vi "glueing_proc_switch_3cartucce.vi"() -> ()   [LabVIEW 2011]
panel:
  in  "Start 3":bool
  in  "spint down - III part":bool
  in  "glue press 2mm - III part":bool
  in  "spint down - III part":bool
  in  "zero Spint for replacing glue 2":bool
  in  "KILL":bool
  in  "PAUSE":bool
  in  "RESUME":bool
  in  "QUIT":bool
  in  "goto y pos":bool
  in  "goto x pos":bool
  in  "Tavolo o stiffback?":bool
  in  "fine tuning y \nmove +2 mm":bool
  in  "fine tuning x \nmove - 2 mm":bool
  in  "fine tuning y \nmove - 2 mm":bool
  in  "fine tuning x \nmove + 2 mm":bool
  in  "Start 2":bool
  in  "spint down - II part":bool
  in  "glue press 2mm - II part":bool
  in  "spint down - II part":bool
  in  "zero done 2":bool
  in  "zero Gluer - end":bool
  in  "zero x - end":bool
  in  "zero y - end":bool
  in  "zero Spint - end":bool
  in  "zero Spint for replacing glue":bool
  in  "spint down 2":bool
  in  "glue press 2mm":bool
  in  "spint down":bool
  in  "Start":bool
  in  "fine tuning z dw 1mm":bool
  in  "fine tuning z up 1mm":bool
  in  "goto z pos 2":bool
  in  "goto z pos":bool
  in  "positioning done":bool
  in  "zero Spint":bool
  out "output":string
  out "command":string
  in  "zero done":bool
  in  "zero Gluer":bool
  in  "zero x":bool
  in  "zero y":bool
  # "In alto: TRUE ---> TAVOLO\nIn basso: FALSE ---> STIFFBACK"
  # "Posiziono in zero"
  # "Vado in posizione"
  # "Fine tuning in posizione x e y \nsolo se necessario"
  # "Muovo spintore e inizio a incollare"
  # "Cambio cartuccia della colla\n\nSTART riprende incollaggio"
  # "Cambio cartuccia della colla\n\nSTART riprende incollaggio"
  # "Scarico la colla e \nritorno a zero"
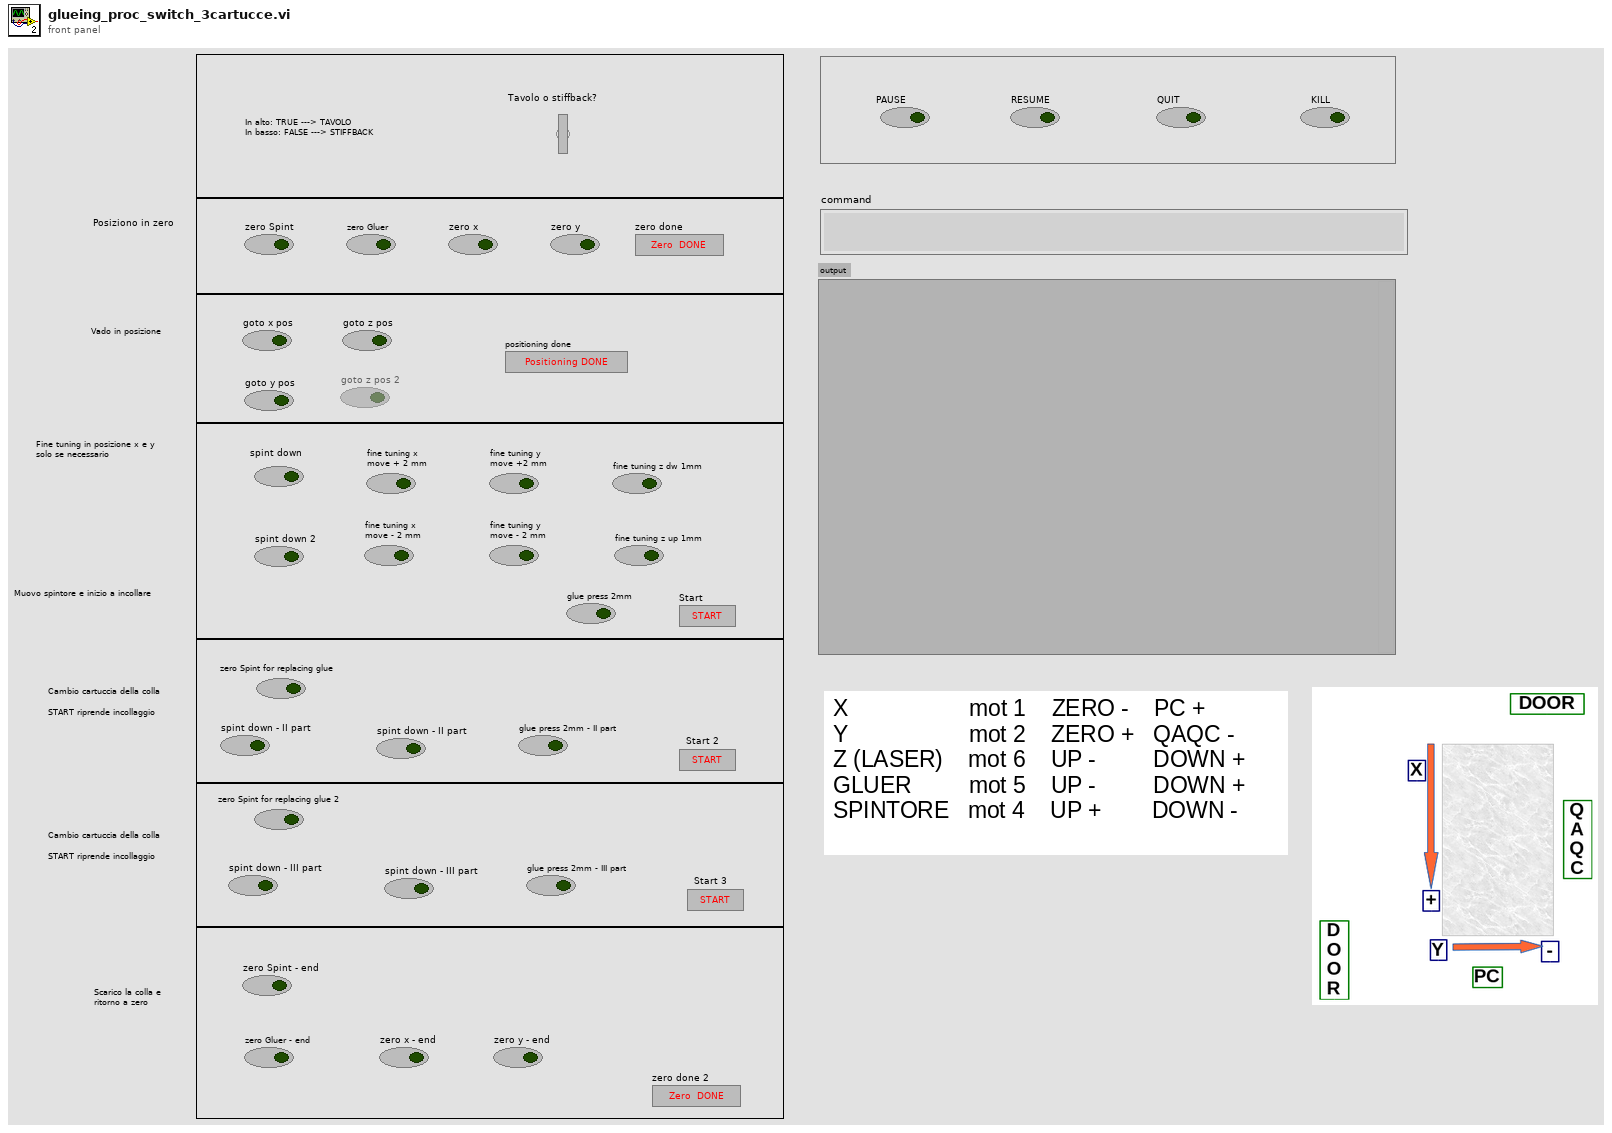
[diagram p1: front panel]
types:
  T1 = enum8{"Enabled", "Disabled", "Disabled and Grayed Out"}
  T2 = enum16{"open", "replace", "create", "open or create", "replace or create", "replace or create with confirmation"}
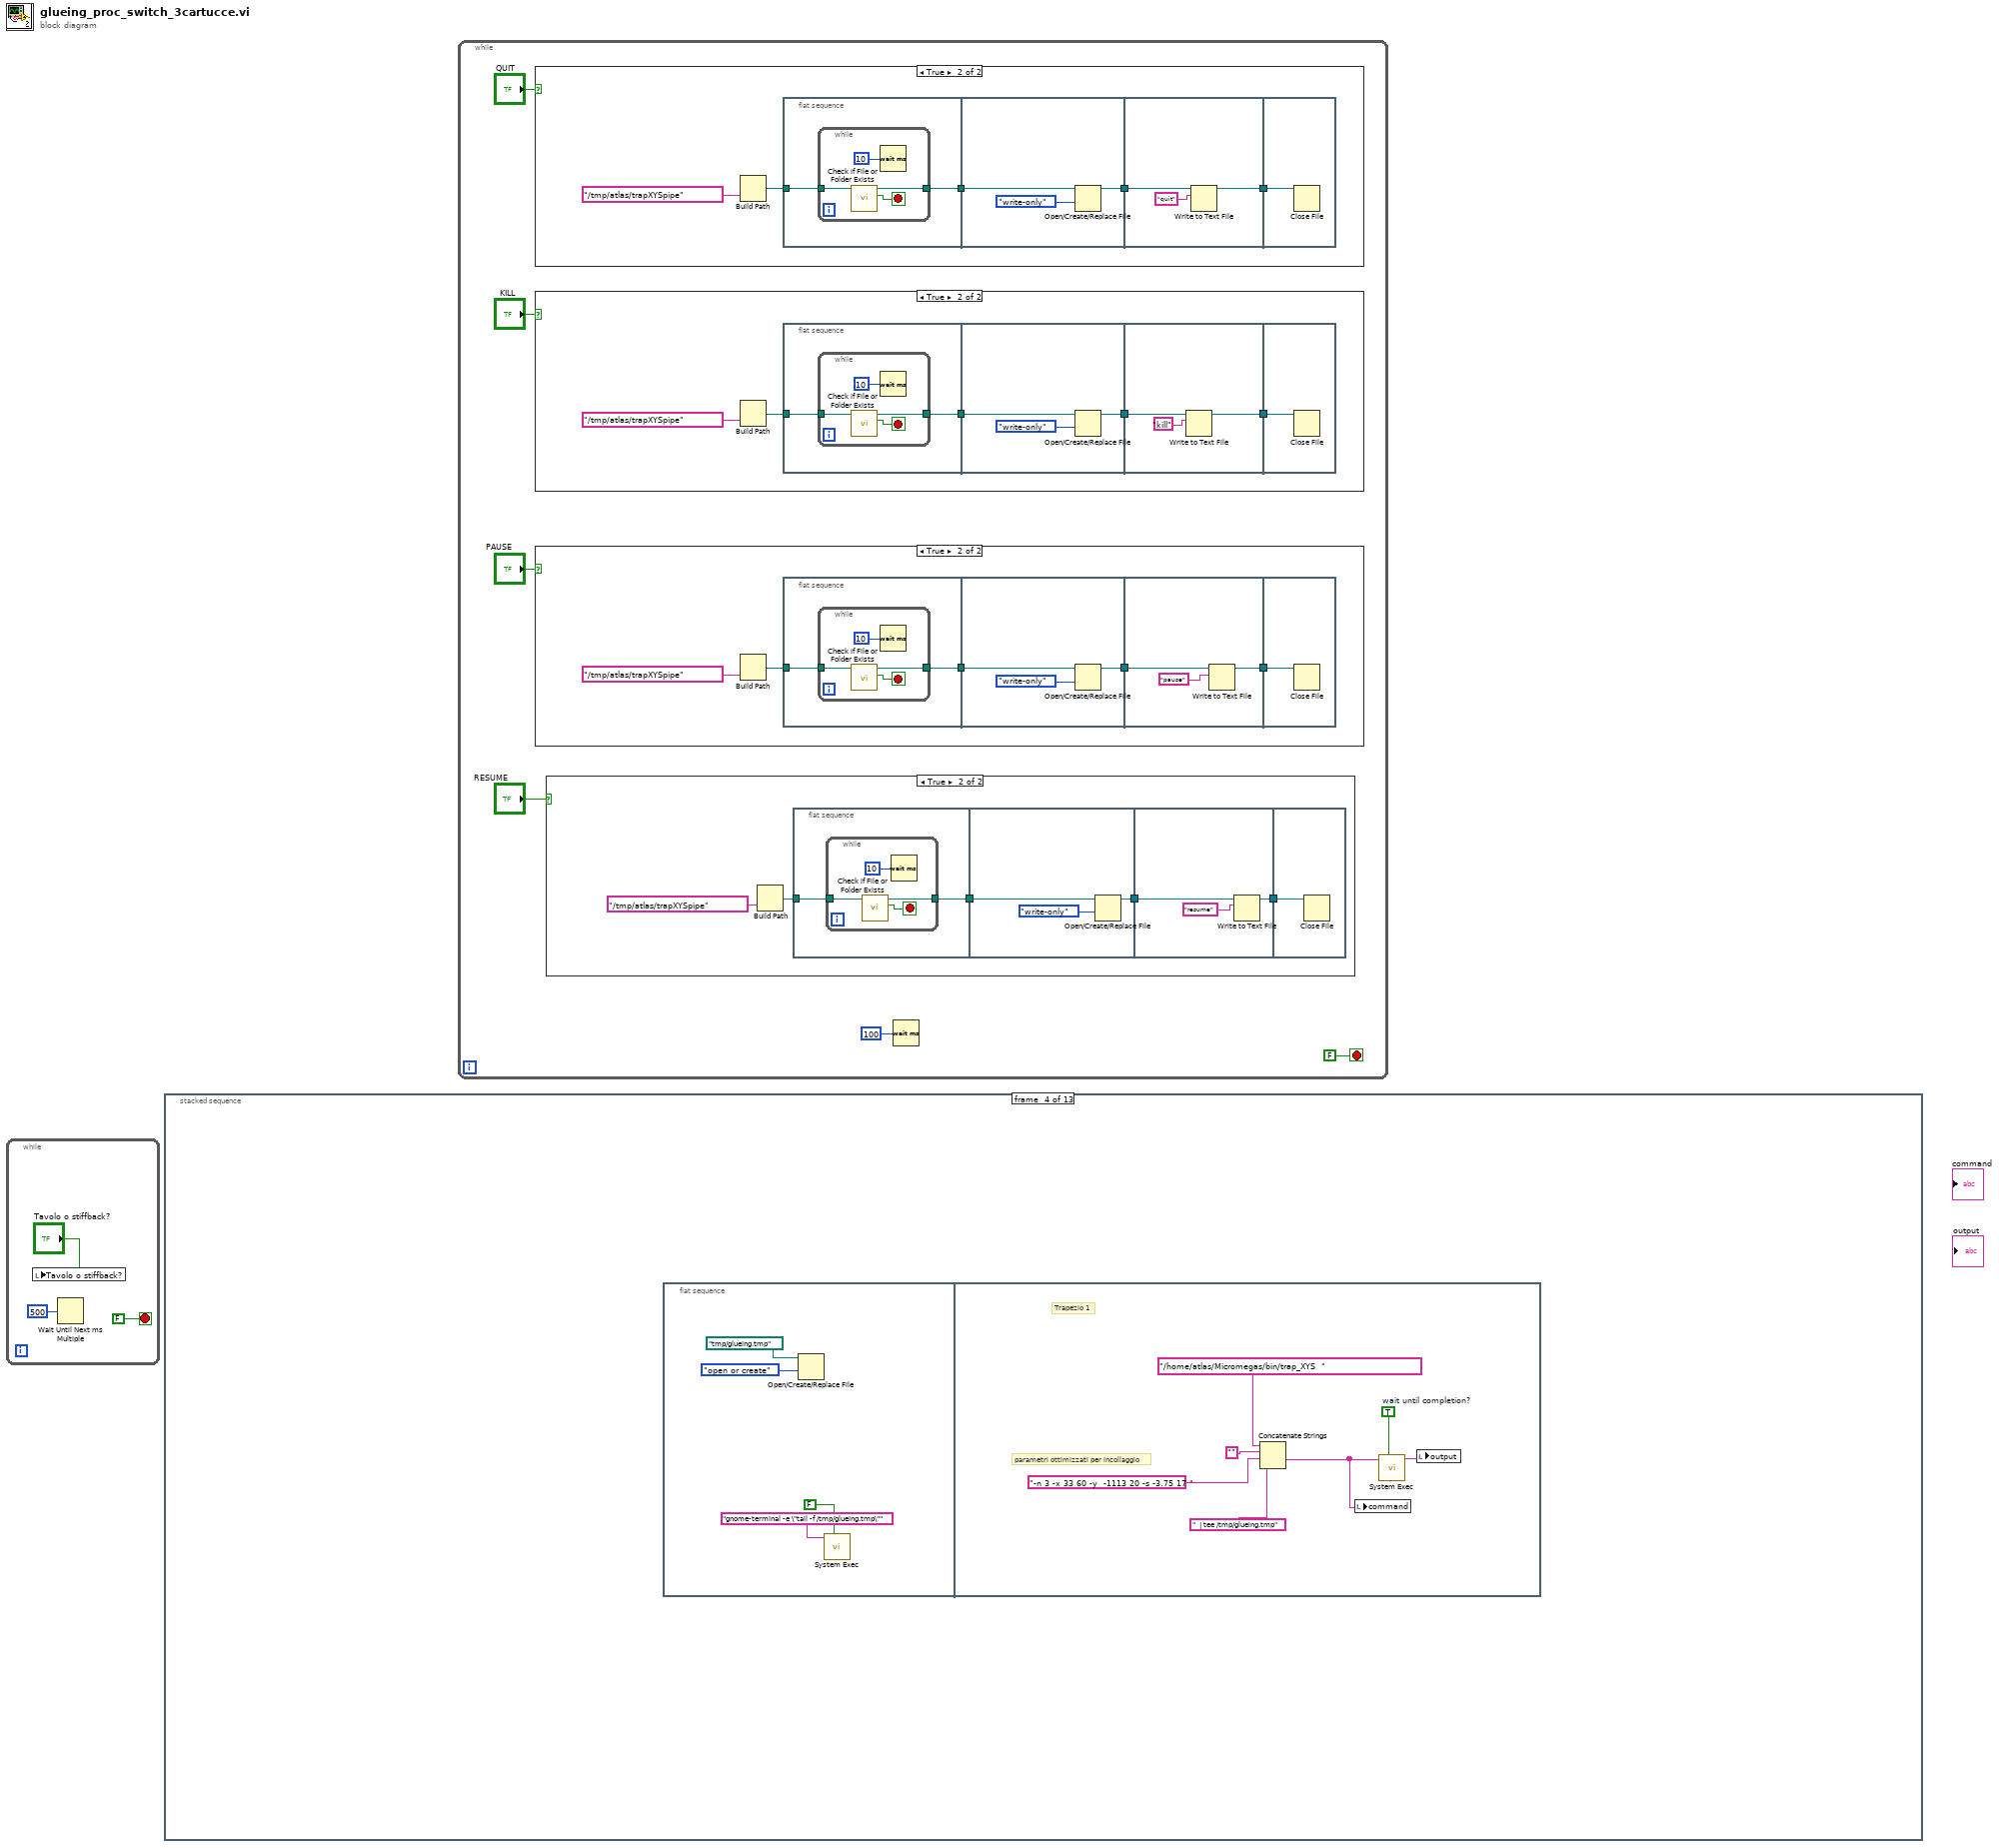
[diagram p0: block diagram]
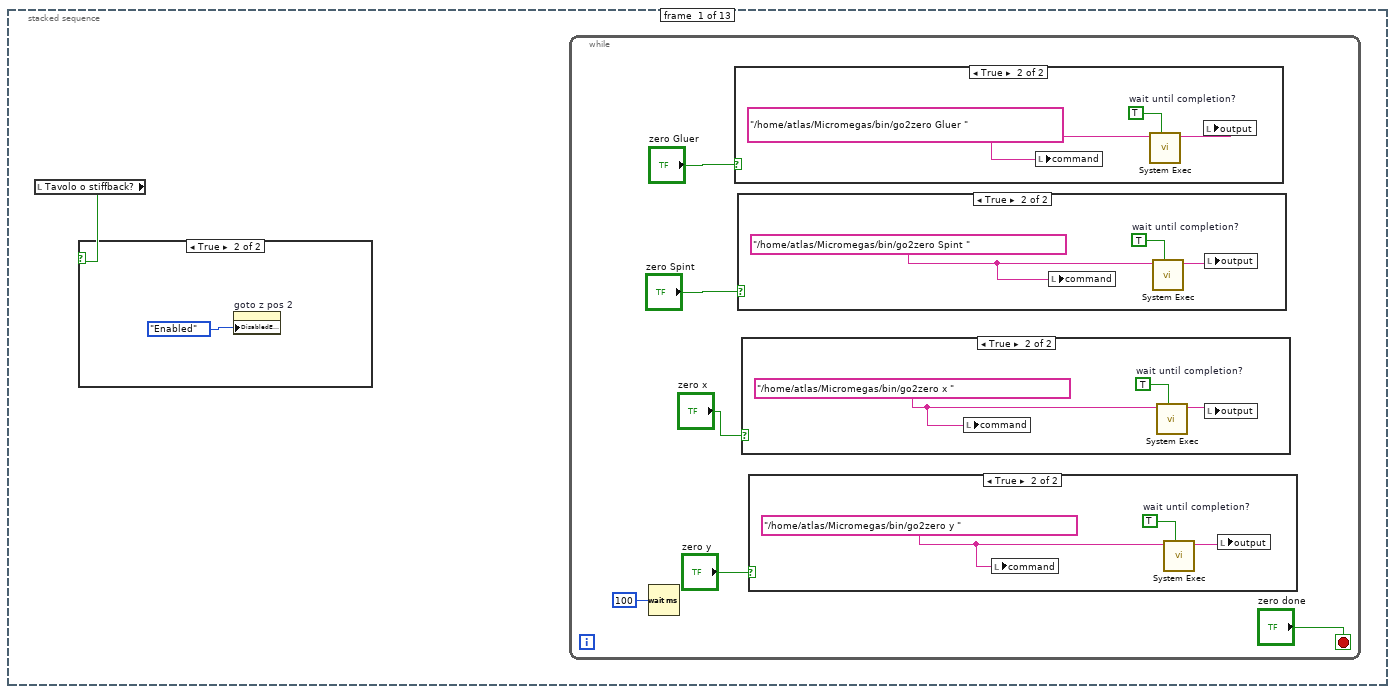
[diagram p6: hidden frame]
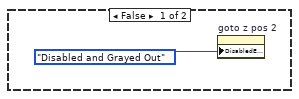
[diagram p7: hidden frame]
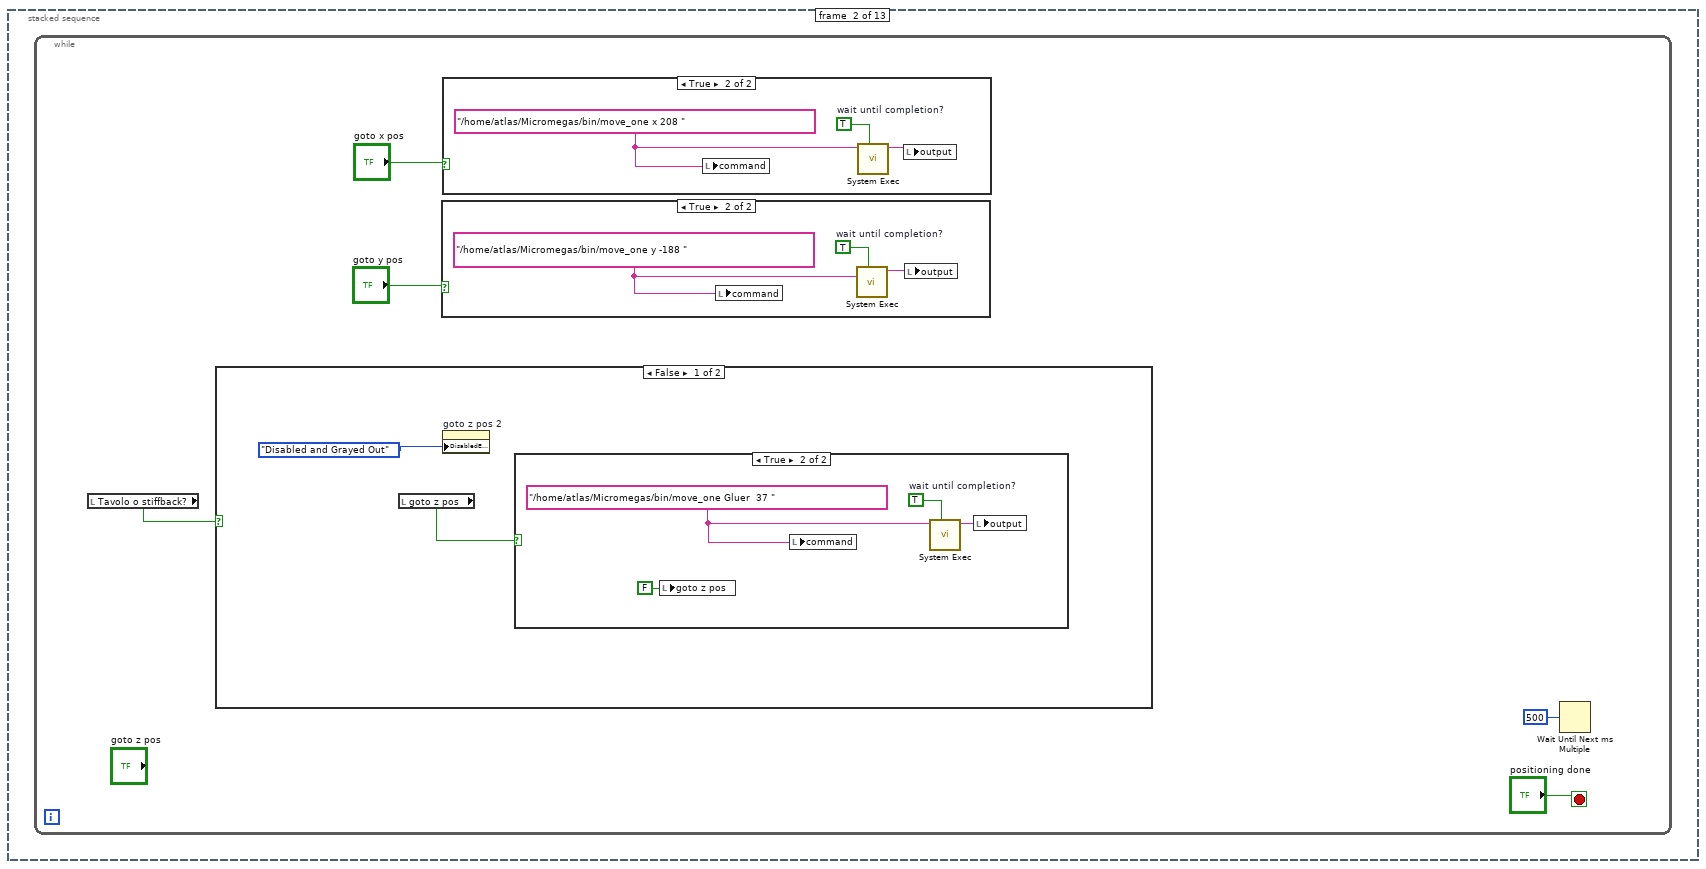
[diagram p12: hidden frame]
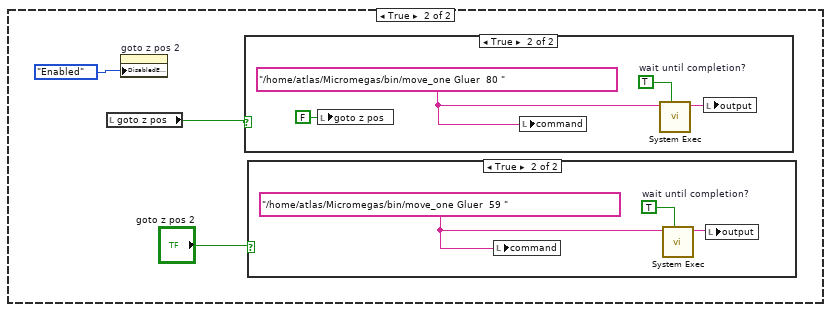
[diagram p14: hidden frame]
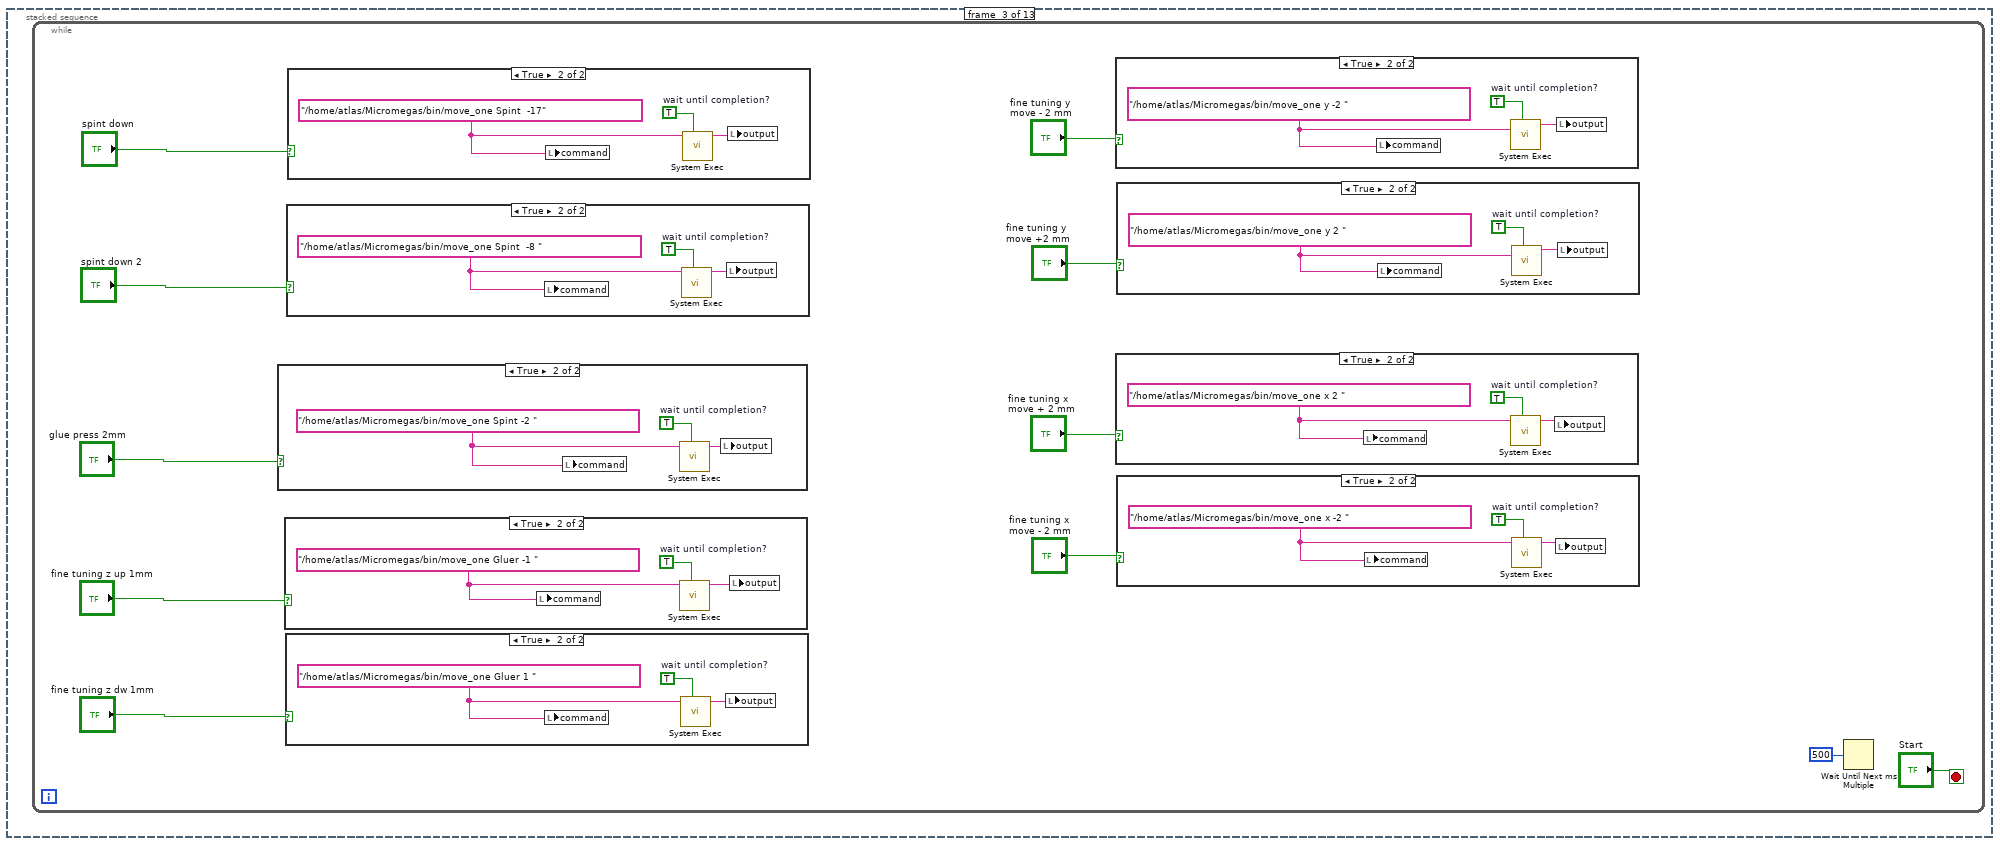
[diagram p19: hidden frame]
diagram:
  n1 = while {
    stop <- FALSE stop-if-true
    n2 = local write "Tavolo o stiffback?"("Tavolo o stiffback?") -> ()
    n3 = Wait Until Next ms Multiple(millisecond multiple=u32 500) -> ()  [unwired: 1 out]
  }
  n4 = stacked-sequence {
    frame #0 {
      n5 = local read "Tavolo o stiffback?"() -> (w4:bool)
      n6 = case shown="True" w4 {
        frame False {
          n7 = property on="goto z pos 2" class="Bool"("DisabledEnum"=T1."Disabled and Grayed Out" ("Disabled")) -> ()  [unwired: 2 in, 2 out]
        }
        frame True {
          n8 = property on="goto z pos 2" class="Bool"("DisabledEnum"=T1."Enabled" ("Disabled")) -> ()  [unwired: 2 in, 2 out]
        }
      }
      n9 = while {
        stop <- "zero done" stop-if-true
        n10 = Wait (ms)(milliseconds to wait=u32 100) -> ()  [unwired: 1 out]
        n11 = case shown="True" "zero Gluer" {
          frame False {
          }
          frame True {
            w23 = "/home/atlas/Micromegas/bin/go2zero Gluer " ("string")
            w24 = TRUE  # wait until completion?
            n12 = local write "command"(w23) -> ()
            n13 = call <vilib>:"System Exec.vi"("wait until completion? (T)"=w24, "command line"=w23) -> ("standard output"=w22:string)  [unwired: 6 in, 3 out]
            n14 = local write "output"(w22) -> ()
          }
        }
        n15 = case shown="True" "zero Spint" {
          frame False {
          }
          frame True {
            w13 = "/home/atlas/Micromegas/bin/go2zero Spint " ("string")
            w15 = TRUE  # wait until completion?
            n16 = local write "command"(w13) -> ()
            n17 = call <vilib>:"System Exec.vi"("wait until completion? (T)"=w15, "command line"=w13) -> ("standard output"=w14:string)  [unwired: 6 in, 3 out]
            n18 = local write "output"(w14) -> ()
          }
        }
        n19 = case shown="True" "zero x" {
          frame False {
          }
          frame True {
            w20 = "/home/atlas/Micromegas/bin/go2zero x " ("string")
            w21 = TRUE  # wait until completion?
            n20 = local write "command"(w20) -> ()
            n21 = call <vilib>:"System Exec.vi"("wait until completion? (T)"=w21, "command line"=w20) -> ("standard output"=w19:string)  [unwired: 6 in, 3 out]
            n22 = local write "output"(w19) -> ()
          }
        }
        n23 = case shown="True" "zero y" {
          frame False {
          }
          frame True {
            w17 = "/home/atlas/Micromegas/bin/go2zero y " ("string")
            w18 = TRUE  # wait until completion?
            n24 = local write "command"(w17) -> ()
            n25 = call <vilib>:"System Exec.vi"("wait until completion? (T)"=w18, "command line"=w17) -> ("standard output"=w16:string)  [unwired: 6 in, 3 out]
            n26 = local write "output"(w16) -> ()
          }
        }
      }
    }
    frame #1 {
      n27 = while {
        stop <- "positioning done" stop-if-true
        n28 = local read "Tavolo o stiffback?"() -> (w25:bool)
        n29 = case shown="False" w25 {
          frame False {
            n30 = local read "goto z pos"() -> (w31:bool)
            n31 = property on="goto z pos 2" class="Bool"("DisabledEnum"=T1."Disabled and Grayed Out" ("Disabled")) -> ()  [unwired: 2 in, 2 out]
            n32 = case shown="True" w31 {
              frame False {
              }
              frame True {
                w33 = "/home/atlas/Micromegas/bin/move_one Gluer  37 " ("string")
                w35 = TRUE  # wait until completion?
                n33 = local write "goto z pos"(FALSE ("goto z pos")) -> ()
                n34 = local write "command"(w33) -> ()
                n35 = call <vilib>:"System Exec.vi"("wait until completion? (T)"=w35, "command line"=w33) -> ("standard output"=w34:string)  [unwired: 6 in, 3 out]
                n36 = local write "output"(w34) -> ()
              }
            }
          }
          frame True {
            n37 = local read "goto z pos"() -> (w37:bool)
            n38 = property on="goto z pos 2" class="Bool"("DisabledEnum"=T1."Enabled" ("Disabled")) -> ()  [unwired: 2 in, 2 out]
            n39 = case shown="True" w37 {
              frame False {
              }
              frame True {
                w43 = "/home/atlas/Micromegas/bin/move_one Gluer  80 " ("string")
                w45 = TRUE  # wait until completion?
                n40 = local write "goto z pos"(FALSE ("goto z pos")) -> ()
                n41 = local write "command"(w43) -> ()
                n42 = call <vilib>:"System Exec.vi"("wait until completion? (T)"=w45, "command line"=w43) -> ("standard output"=w44:string)  [unwired: 6 in, 3 out]
                n43 = local write "output"(w44) -> ()
              }
            }
            n44 = case shown="True" "goto z pos 2" {
              frame False {
              }
              frame True {
                w39 = "/home/atlas/Micromegas/bin/move_one Gluer  59 " ("string")
                w41 = TRUE  # wait until completion?
                n45 = local write "command"(w39) -> ()
                n46 = call <vilib>:"System Exec.vi"("wait until completion? (T)"=w41, "command line"=w39) -> ("standard output"=w40:string)  [unwired: 6 in, 3 out]
                n47 = local write "output"(w40) -> ()
              }
            }
          }
        }
        n48 = case shown="True" "goto y pos" {
          frame False {
          }
          frame True {
            w46 = "/home/atlas/Micromegas/bin/move_one y -188 " ("string")
            w48 = TRUE  # wait until completion?
            n49 = local write "command"(w46) -> ()
            n50 = call <vilib>:"System Exec.vi"("wait until completion? (T)"=w48, "command line"=w46) -> ("standard output"=w47:string)  [unwired: 6 in, 3 out]
            n51 = local write "output"(w47) -> ()
          }
        }
        n52 = case shown="True" "goto x pos" {
          frame False {
          }
          frame True {
            w49 = "/home/atlas/Micromegas/bin/move_one x 208 " ("string")
            w51 = TRUE  # wait until completion?
            n53 = local write "command"(w49) -> ()
            n54 = call <vilib>:"System Exec.vi"("wait until completion? (T)"=w51, "command line"=w49) -> ("standard output"=w50:string)  [unwired: 6 in, 3 out]
            n55 = local write "output"(w50) -> ()
          }
        }
        n56 = Wait Until Next ms Multiple(millisecond multiple=u32 500) -> ()  [unwired: 1 out]
      }
    }
    frame #2 {
      n57 = while {
        stop <- "Start" stop-if-true
        n58 = case shown="True" "glue press 2mm" {
          frame False {
          }
          frame True {
            w85 = "/home/atlas/Micromegas/bin/move_one Spint -2 " ("string")
            w86 = TRUE  # wait until completion?
            n59 = local write "command"(w85) -> ()
            n60 = call <vilib>:"System Exec.vi"("wait until completion? (T)"=w86, "command line"=w85) -> ("standard output"=w84:string)  [unwired: 6 in, 3 out]
            n61 = local write "output"(w84) -> ()
          }
        }
        n62 = case shown="True" "fine tuning z up 1mm" {
          frame False {
          }
          frame True {
            w66 = "/home/atlas/Micromegas/bin/move_one Gluer -1 " ("string")
            w68 = TRUE  # wait until completion?
            n63 = local write "command"(w66) -> ()
            n64 = call <vilib>:"System Exec.vi"("wait until completion? (T)"=w68, "command line"=w66) -> ("standard output"=w67:string)  [unwired: 6 in, 3 out]
            n65 = local write "output"(w67) -> ()
          }
        }
        n66 = case shown="True" "fine tuning z dw 1mm" {
          frame False {
          }
          frame True {
            w63 = "/home/atlas/Micromegas/bin/move_one Gluer 1 " ("string")
            w65 = TRUE  # wait until completion?
            n67 = local write "command"(w63) -> ()
            n68 = call <vilib>:"System Exec.vi"("wait until completion? (T)"=w65, "command line"=w63) -> ("standard output"=w64:string)  [unwired: 6 in, 3 out]
            n69 = local write "output"(w64) -> ()
          }
        }
        n70 = case shown="True" "spint down 2" {
          frame False {
          }
          frame True {
            w81 = "/home/atlas/Micromegas/bin/move_one Spint  -8 " ("string")
            w83 = TRUE  # wait until completion?
            n71 = local write "command"(w81) -> ()
            n72 = call <vilib>:"System Exec.vi"("wait until completion? (T)"=w83, "command line"=w81) -> ("standard output"=w82:string)  [unwired: 6 in, 3 out]
            n73 = local write "output"(w82) -> ()
          }
        }
        n74 = case shown="True" "spint down" {
          frame False {
          }
          frame True {
            w87 = "/home/atlas/Micromegas/bin/move_one Spint  -17" ("string")
            w89 = TRUE  # wait until completion?
            n75 = local write "command"(w87) -> ()
            n76 = call <vilib>:"System Exec.vi"("wait until completion? (T)"=w89, "command line"=w87) -> ("standard output"=w88:string)  [unwired: 6 in, 3 out]
            n77 = local write "output"(w88) -> ()
          }
        }
        n78 = case shown="True" "fine tuning y \nmove - 2 mm" {
          frame False {
          }
          frame True {
            w78 = "/home/atlas/Micromegas/bin/move_one y -2 " ("string")
            w80 = TRUE  # wait until completion?
            n79 = local write "command"(w78) -> ()
            n80 = call <vilib>:"System Exec.vi"("wait until completion? (T)"=w80, "command line"=w78) -> ("standard output"=w79:string)  [unwired: 6 in, 3 out]
            n81 = local write "output"(w79) -> ()
          }
        }
        n82 = case shown="True" "fine tuning x \nmove + 2 mm" {
          frame False {
          }
          frame True {
            w72 = "/home/atlas/Micromegas/bin/move_one x 2 " ("string")
            w74 = TRUE  # wait until completion?
            n83 = local write "command"(w72) -> ()
            n84 = call <vilib>:"System Exec.vi"("wait until completion? (T)"=w74, "command line"=w72) -> ("standard output"=w73:string)  [unwired: 6 in, 3 out]
            n85 = local write "output"(w73) -> ()
          }
        }
        n86 = case shown="True" "fine tuning y \nmove +2 mm" {
          frame False {
          }
          frame True {
            w75 = "/home/atlas/Micromegas/bin/move_one y 2 " ("string")
            w77 = TRUE  # wait until completion?
            n87 = local write "command"(w75) -> ()
            n88 = call <vilib>:"System Exec.vi"("wait until completion? (T)"=w77, "command line"=w75) -> ("standard output"=w76:string)  [unwired: 6 in, 3 out]
            n89 = local write "output"(w76) -> ()
          }
        }
        n90 = case shown="True" "fine tuning x \nmove - 2 mm" {
          frame False {
          }
          frame True {
            w69 = "/home/atlas/Micromegas/bin/move_one x -2 " ("string")
            w71 = TRUE  # wait until completion?
            n91 = local write "command"(w69) -> ()
            n92 = call <vilib>:"System Exec.vi"("wait until completion? (T)"=w71, "command line"=w69) -> ("standard output"=w70:string)  [unwired: 6 in, 3 out]
            n93 = local write "output"(w70) -> ()
          }
        }
        n94 = Wait Until Next ms Multiple(millisecond multiple=u32 500) -> ()  [unwired: 1 out]
      }
    }
    frame #3 {
      n95 = flat-sequence {
        frame #0 {
          n96 = Open/Create/Replace File(file path (use dialog)=path "/tmp/glueing.tmp", operation (0:open)=T2."open or create") -> ()  [unwired: 4 in, 3 out]
          n97 = call <vilib>:"System Exec.vi"("wait until completion? (T)"=FALSE, "command line"="gnome-terminal -e \"tail -f /tmp/glueing.tmp\"" ("logwindow")) -> ()  [unwired: 6 in, 4 out]
        }
        frame #1 {
          w100 = TRUE  # wait until completion?
          # "Trapezio 1"
          # "parametri ottimizzati per incollaggio"
          n98 = Concatenate Strings("/home/atlas/Micromegas/bin/trap_XYS  " ("string"), "" ("string"), "-n 3 -x 33 60 -y  -1113 20 -s -3.75 17 " ("string"), "  | tee /tmp/glueing.tmp" ("string")) -> (w95:string)
          n99 = local write "command"(w95) -> ()
          n100 = call <vilib>:"System Exec.vi"("wait until completion? (T)"=w100, "command line"=w95) -> ("standard output"=w94:string)  [unwired: 6 in, 3 out]
          n101 = local write "output"(w94) -> ()
        }
      }
    }
    frame #4 {
      n102 = while {
        stop <- w102 stop-if-true
        n103 = case shown="True" "zero Spint for replacing glue" {
          tunnel: [FALSE TRUE] -> w102
          frame False {
          }
          frame True {
            w106 = "/home/atlas/Micromegas/bin/go2zero Spint " ("string")
            w108 = TRUE  # wait until completion?
            n104 = local write "command"(w106) -> ()
            n105 = call <vilib>:"System Exec.vi"("wait until completion? (T)"=w108, "command line"=w106) -> ("standard output"=w107:string)  [unwired: 6 in, 3 out]
            n106 = local write "output"(w107) -> ()
          }
        }
        n107 = Wait (ms)(milliseconds to wait=u32 100) -> ()  [unwired: 1 out]
      }
    }
    frame #5 {
      n108 = One Button Dialog(message="Replace the glue!\nPress OK after done") -> ()  [unwired: 1 in, 1 out]
    }
    frame #6 {
      n109 = while {
        stop <- "Start 2" stop-if-true
        n110 = case shown="True" "glue press 2mm - II part" {
          frame False {
          }
          frame True {
            w119 = "/home/atlas/Micromegas/bin/move_one Spint -2 " ("string")
            w120 = TRUE  # wait until completion?
            n111 = local write "command"(w119) -> ()
            n112 = call <vilib>:"System Exec.vi"("wait until completion? (T)"=w120, "command line"=w119) -> ("standard output"=w118:string)  [unwired: 6 in, 3 out]
            n113 = local write "output"(w118) -> ()
          }
        }
        n114 = case shown="True" "spint down - II part" {
          frame False {
          }
          frame True {
            w115 = "/home/atlas/Micromegas/bin/move_one Spint  -8 " ("string")
            w117 = TRUE  # wait until completion?
            n115 = local write "command"(w115) -> ()
            n116 = call <vilib>:"System Exec.vi"("wait until completion? (T)"=w117, "command line"=w115) -> ("standard output"=w116:string)  [unwired: 6 in, 3 out]
            n117 = local write "output"(w116) -> ()
          }
        }
        n118 = case shown="True" "spint down - II part" {
          frame False {
          }
          frame True {
            w121 = "/home/atlas/Micromegas/bin/move_one Spint  -17" ("string")
            w123 = TRUE  # wait until completion?
            n119 = local write "command"(w121) -> ()
            n120 = call <vilib>:"System Exec.vi"("wait until completion? (T)"=w123, "command line"=w121) -> ("standard output"=w122:string)  [unwired: 6 in, 3 out]
            n121 = local write "output"(w122) -> ()
          }
        }
        n122 = Wait Until Next ms Multiple(millisecond multiple=u32 500) -> ()  [unwired: 1 out]
      }
    }
    frame #7 {
      n123 = flat-sequence {
        frame #0 {
          n124 = Open/Create/Replace File(file path (use dialog)=path "/tmp/glueing.tmp", operation (0:open)=T2."open or create") -> ()  [unwired: 4 in, 3 out]
          n125 = call <vilib>:"System Exec.vi"("wait until completion? (T)"=FALSE, "command line"="gnome-terminal -e \"tail -f /tmp/glueing.tmp\"" ("logwindow")) -> ()  [unwired: 6 in, 4 out]
        }
        frame #1 {
          w134 = TRUE  # wait until completion?
          # "Trapezio 2"
          # "parametri ottimizzati per incollaggio"
          n126 = Concatenate Strings("/home/atlas/Micromegas/bin/trap_XYS  " ("string"), "" ("string"), "-n 20 -x 33 60 -y  -1016 20 -s -3.45 17 " ("string"), "  | tee /tmp/glueing.tmp" ("string")) -> (w129:string)
          n127 = local write "command"(w129) -> ()
          n128 = call <vilib>:"System Exec.vi"("wait until completion? (T)"=w134, "command line"=w129) -> ("standard output"=w128:string)  [unwired: 6 in, 3 out]
          n129 = local write "output"(w128) -> ()
        }
      }
    }
    frame #8 {
      n130 = while {
        stop <- w136 stop-if-true
        n131 = case shown="True" "zero Spint for replacing glue 2" {
          tunnel: [FALSE TRUE] -> w136
          frame False {
          }
          frame True {
            w140 = "/home/atlas/Micromegas/bin/go2zero Spint " ("string")
            w142 = TRUE  # wait until completion?
            n132 = local write "command"(w140) -> ()
            n133 = call <vilib>:"System Exec.vi"("wait until completion? (T)"=w142, "command line"=w140) -> ("standard output"=w141:string)  [unwired: 6 in, 3 out]
            n134 = local write "output"(w141) -> ()
          }
        }
        n135 = Wait (ms)(milliseconds to wait=u32 100) -> ()  [unwired: 1 out]
      }
    }
    frame #9 {
      n136 = One Button Dialog(message="Replace the glue!\nPress OK after done") -> ()  [unwired: 1 in, 1 out]
    }
    frame #10 {
      n137 = while {
        stop <- "Start 3" stop-if-true
        n138 = case shown="True" "glue press 2mm - III part" {
          frame False {
          }
          frame True {
            w153 = "/home/atlas/Micromegas/bin/move_one Spint -2 " ("string")
            w154 = TRUE  # wait until completion?
            n139 = local write "command"(w153) -> ()
            n140 = call <vilib>:"System Exec.vi"("wait until completion? (T)"=w154, "command line"=w153) -> ("standard output"=w152:string)  [unwired: 6 in, 3 out]
            n141 = local write "output"(w152) -> ()
          }
        }
        n142 = case shown="True" "spint down - III part" {
          frame False {
          }
          frame True {
            w149 = "/home/atlas/Micromegas/bin/move_one Spint  -8 " ("string")
            w151 = TRUE  # wait until completion?
            n143 = local write "command"(w149) -> ()
            n144 = call <vilib>:"System Exec.vi"("wait until completion? (T)"=w151, "command line"=w149) -> ("standard output"=w150:string)  [unwired: 6 in, 3 out]
            n145 = local write "output"(w150) -> ()
          }
        }
        n146 = case shown="True" "spint down - III part" {
          frame False {
          }
          frame True {
            w155 = "/home/atlas/Micromegas/bin/move_one Spint  -17" ("string")
            w157 = TRUE  # wait until completion?
            n147 = local write "command"(w155) -> ()
            n148 = call <vilib>:"System Exec.vi"("wait until completion? (T)"=w157, "command line"=w155) -> ("standard output"=w156:string)  [unwired: 6 in, 3 out]
            n149 = local write "output"(w156) -> ()
          }
        }
        n150 = Wait Until Next ms Multiple(millisecond multiple=u32 500) -> ()  [unwired: 1 out]
      }
    }
    frame #11 {
      n151 = flat-sequence {
        frame #0 {
          n152 = Open/Create/Replace File(file path (use dialog)=path "/tmp/glueing.tmp", operation (0:open)=T2."open or create") -> ()  [unwired: 4 in, 3 out]
          n153 = call <vilib>:"System Exec.vi"("wait until completion? (T)"=FALSE, "command line"="gnome-terminal -e \"tail -f /tmp/glueing.tmp\"" ("logwindow")) -> ()  [unwired: 6 in, 4 out]
        }
        frame #1 {
          w168 = TRUE  # wait until completion?
          # "Trapezio 2"
          # "parametri ottimizzati per incollaggio"
          n154 = Concatenate Strings("/home/atlas/Micromegas/bin/trap_XYS  " ("string"), "" ("string"), "-n 31 -x 33 60 -y  -770 20 -s -2.6 17 " ("string"), "  | tee /tmp/glueing.tmp" ("string")) -> (w163:string)
          n155 = local write "command"(w163) -> ()
          n156 = call <vilib>:"System Exec.vi"("wait until completion? (T)"=w168, "command line"=w163) -> ("standard output"=w162:string)  [unwired: 6 in, 3 out]
          n157 = local write "output"(w162) -> ()
        }
      }
    }
    frame #12 {
      n158 = while {
        stop <- "zero done 2" stop-if-true
        n159 = Wait (ms)(milliseconds to wait=u32 100) -> ()  [unwired: 1 out]
        n160 = case shown="True" "zero Gluer - end" {
          frame False {
          }
          frame True {
            w185 = "/home/atlas/Micromegas/bin/go2zero Gluer " ("string")
            w186 = TRUE  # wait until completion?
            n161 = local write "command"(w185) -> ()
            n162 = call <vilib>:"System Exec.vi"("wait until completion? (T)"=w186, "command line"=w185) -> ("standard output"=w184:string)  [unwired: 6 in, 3 out]
            n163 = local write "output"(w184) -> ()
          }
        }
        n164 = case shown="True" "zero Spint - end" {
          frame False {
          }
          frame True {
            w175 = "/home/atlas/Micromegas/bin/go2zero Spint " ("string")
            w177 = TRUE  # wait until completion?
            n165 = local write "command"(w175) -> ()
            n166 = call <vilib>:"System Exec.vi"("wait until completion? (T)"=w177, "command line"=w175) -> ("standard output"=w176:string)  [unwired: 6 in, 3 out]
            n167 = local write "output"(w176) -> ()
          }
        }
        n168 = case shown="True" "zero x - end" {
          frame False {
          }
          frame True {
            w182 = "/home/atlas/Micromegas/bin/go2zero x " ("string")
            w183 = TRUE  # wait until completion?
            n169 = local write "command"(w182) -> ()
            n170 = call <vilib>:"System Exec.vi"("wait until completion? (T)"=w183, "command line"=w182) -> ("standard output"=w181:string)  [unwired: 6 in, 3 out]
            n171 = local write "output"(w181) -> ()
          }
        }
        n172 = case shown="True" "zero y - end" {
          frame False {
          }
          frame True {
            w179 = "/home/atlas/Micromegas/bin/go2zero y " ("string")
            w180 = TRUE  # wait until completion?
            n173 = local write "command"(w179) -> ()
            n174 = call <vilib>:"System Exec.vi"("wait until completion? (T)"=w180, "command line"=w179) -> ("standard output"=w178:string)  [unwired: 6 in, 3 out]
            n175 = local write "output"(w178) -> ()
          }
        }
      }
    }
  }
  n176 = while {
    stop <- FALSE stop-if-true
    n177 = case shown="True" "QUIT" {
      frame False {
      }
      frame True {
        n178 = Build Path(name or relative path="/tmp/atlas/trapXYSpipe" ("string")) -> (appended path=w247:path)  [unwired: 1 in]
        n179 = flat-sequence {
          tunnel: [w253] -> w251
          tunnel: w247 -> [w252]
          tunnel: w251 -> [w260]
          tunnel: [w258] -> w250
          tunnel: w250 -> [w263]
          tunnel: [w262] -> w249
          tunnel: w249 -> [w264]
          frame #0 {
            n180 = while {
              tunnel: [w255] -> w253
              tunnel: w252 -> [w254]
              stop <- w256 stop-if-true
              n181 = call <vilib>:"Check if File or Folder Exists.vi"("path"=w254) -> ("file or folder exists?"=w256:bool, "dup path"=w255:path)  [unwired: 8 in, 1 out]
              n182 = Wait (ms)(milliseconds to wait=u32 10) -> ()  [unwired: 1 out]
            }
          }
          frame #1 {
            n183 = Open/Create/Replace File(file path (use dialog)=w260, access (0:read/write)=enum16{"read/write", "read-only", "write-only"}."write-only") -> (refnum out=w258:refnum<file>)  [unwired: 4 in, 2 out]
          }
          frame #2 {
            n184 = Write to Text File(file (use dialog)=w263, text="quit") -> (refnum out=w262:refnum<file>)  [unwired: 2 in, 2 out]
          }
          frame #3 {
            n185 = Close File(refnum=w264) -> ()  [unwired: 1 in, 2 out]
          }
        }
      }
    }
    n186 = case shown="True" "KILL" {
      frame False {
      }
      frame True {
        n187 = Build Path(name or relative path="/tmp/atlas/trapXYSpipe" ("string")) -> (appended path=w211:path)  [unwired: 1 in]
        n188 = flat-sequence {
          tunnel: [w217] -> w215
          tunnel: w211 -> [w216]
          tunnel: w215 -> [w224]
          tunnel: [w222] -> w214
          tunnel: w214 -> [w227]
          tunnel: [w226] -> w213
          tunnel: w213 -> [w228]
          frame #0 {
            n189 = while {
              tunnel: [w219] -> w217
              tunnel: w216 -> [w218]
              stop <- w220 stop-if-true
              n190 = call <vilib>:"Check if File or Folder Exists.vi"("path"=w218) -> ("file or folder exists?"=w220:bool, "dup path"=w219:path)  [unwired: 8 in, 1 out]
              n191 = Wait (ms)(milliseconds to wait=u32 10) -> ()  [unwired: 1 out]
            }
          }
          frame #1 {
            n192 = Open/Create/Replace File(file path (use dialog)=w224, access (0:read/write)=enum16{"read/write", "read-only", "write-only"}."write-only") -> (refnum out=w222:refnum<file>)  [unwired: 4 in, 2 out]
          }
          frame #2 {
            n193 = Write to Text File(file (use dialog)=w227, text="kill") -> (refnum out=w226:refnum<file>)  [unwired: 2 in, 2 out]
          }
          frame #3 {
            n194 = Close File(refnum=w228) -> ()  [unwired: 1 in, 2 out]
          }
        }
      }
    }
    n195 = case shown="True" "PAUSE" {
      frame False {
      }
      frame True {
        n196 = Build Path(name or relative path="/tmp/atlas/trapXYSpipe" ("string")) -> (appended path=w193:path)  [unwired: 1 in]
        n197 = flat-sequence {
          tunnel: [w199] -> w197
          tunnel: w193 -> [w198]
          tunnel: w197 -> [w206]
          tunnel: [w204] -> w196
          tunnel: w196 -> [w209]
          tunnel: [w208] -> w195
          tunnel: w195 -> [w210]
          frame #0 {
            n198 = while {
              tunnel: [w201] -> w199
              tunnel: w198 -> [w200]
              stop <- w202 stop-if-true
              n199 = call <vilib>:"Check if File or Folder Exists.vi"("path"=w200) -> ("file or folder exists?"=w202:bool, "dup path"=w201:path)  [unwired: 8 in, 1 out]
              n200 = Wait (ms)(milliseconds to wait=u32 10) -> ()  [unwired: 1 out]
            }
          }
          frame #1 {
            n201 = Open/Create/Replace File(file path (use dialog)=w206, access (0:read/write)=enum16{"read/write", "read-only", "write-only"}."write-only") -> (refnum out=w204:refnum<file>)  [unwired: 4 in, 2 out]
          }
          frame #2 {
            n202 = Write to Text File(file (use dialog)=w209, text="pause") -> (refnum out=w208:refnum<file>)  [unwired: 2 in, 2 out]
          }
          frame #3 {
            n203 = Close File(refnum=w210) -> ()  [unwired: 1 in, 2 out]
          }
        }
      }
    }
    n204 = case shown="True" "RESUME" {
      frame False {
      }
      frame True {
        n205 = Build Path(name or relative path="/tmp/atlas/trapXYSpipe" ("string")) -> (appended path=w229:path)  [unwired: 1 in]
        n206 = flat-sequence {
          tunnel: [w235] -> w233
          tunnel: w229 -> [w234]
          tunnel: w233 -> [w242]
          tunnel: [w240] -> w232
          tunnel: w232 -> [w245]
          tunnel: [w244] -> w231
          tunnel: w231 -> [w246]
          frame #0 {
            n207 = while {
              tunnel: [w237] -> w235
              tunnel: w234 -> [w236]
              stop <- w238 stop-if-true
              n208 = call <vilib>:"Check if File or Folder Exists.vi"("path"=w236) -> ("file or folder exists?"=w238:bool, "dup path"=w237:path)  [unwired: 8 in, 1 out]
              n209 = Wait (ms)(milliseconds to wait=u32 10) -> ()  [unwired: 1 out]
            }
          }
          frame #1 {
            n210 = Open/Create/Replace File(file path (use dialog)=w242, access (0:read/write)=enum16{"read/write", "read-only", "write-only"}."write-only") -> (refnum out=w240:refnum<file>)  [unwired: 4 in, 2 out]
          }
          frame #2 {
            n211 = Write to Text File(file (use dialog)=w245, text="resume") -> (refnum out=w244:refnum<file>)  [unwired: 2 in, 2 out]
          }
          frame #3 {
            n212 = Close File(refnum=w246) -> ()  [unwired: 1 in, 2 out]
          }
        }
      }
    }
    n213 = Wait (ms)(milliseconds to wait=100) -> ()  [unwired: 1 out]
  }
